vi "Get Bus A Data.vi"(5 "Component ID":u8, 7 "FPGA Interface":refnum<class "FPGA Interface.lvclass">, 8 "error in (no error)":errorcluster, 11 "Bus Monitor in":refnum<class "Bus Monitor.lvclass">) -> (0 "error out":errorcluster, 3 "Bus Monitor out":refnum<class "Bus Monitor.lvclass">)   [LabVIEW 2020, in "BCI-1553 API.lvlib" / "Bus Monitor.lvclass"]
doc: "Retrieves the entire command list for Bus A and parses out a list of command words and data pointer words that are resorted into chronological order."
uses:
  Bus Monitor.lvclass
  Dependencies/FPGA Interface/FPGA Interface.lvclass
  Bus Monitor.lvclass/Bus Monitor.ctl
  Dependencies/Registry/Registry.lvclass/Registry.ctl
  Dependencies/Registry/Registry.lvclass
panel:
  out "Data 2":u16=1 format="%.0x"
  out "Data 1":u16=1 format="%.0x"
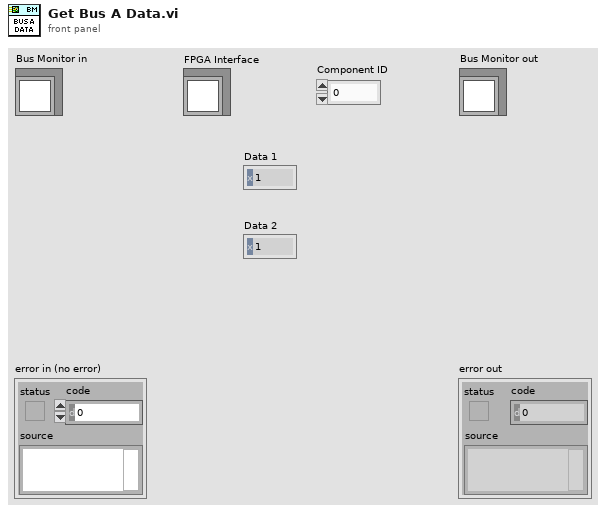
[diagram p1: front panel]
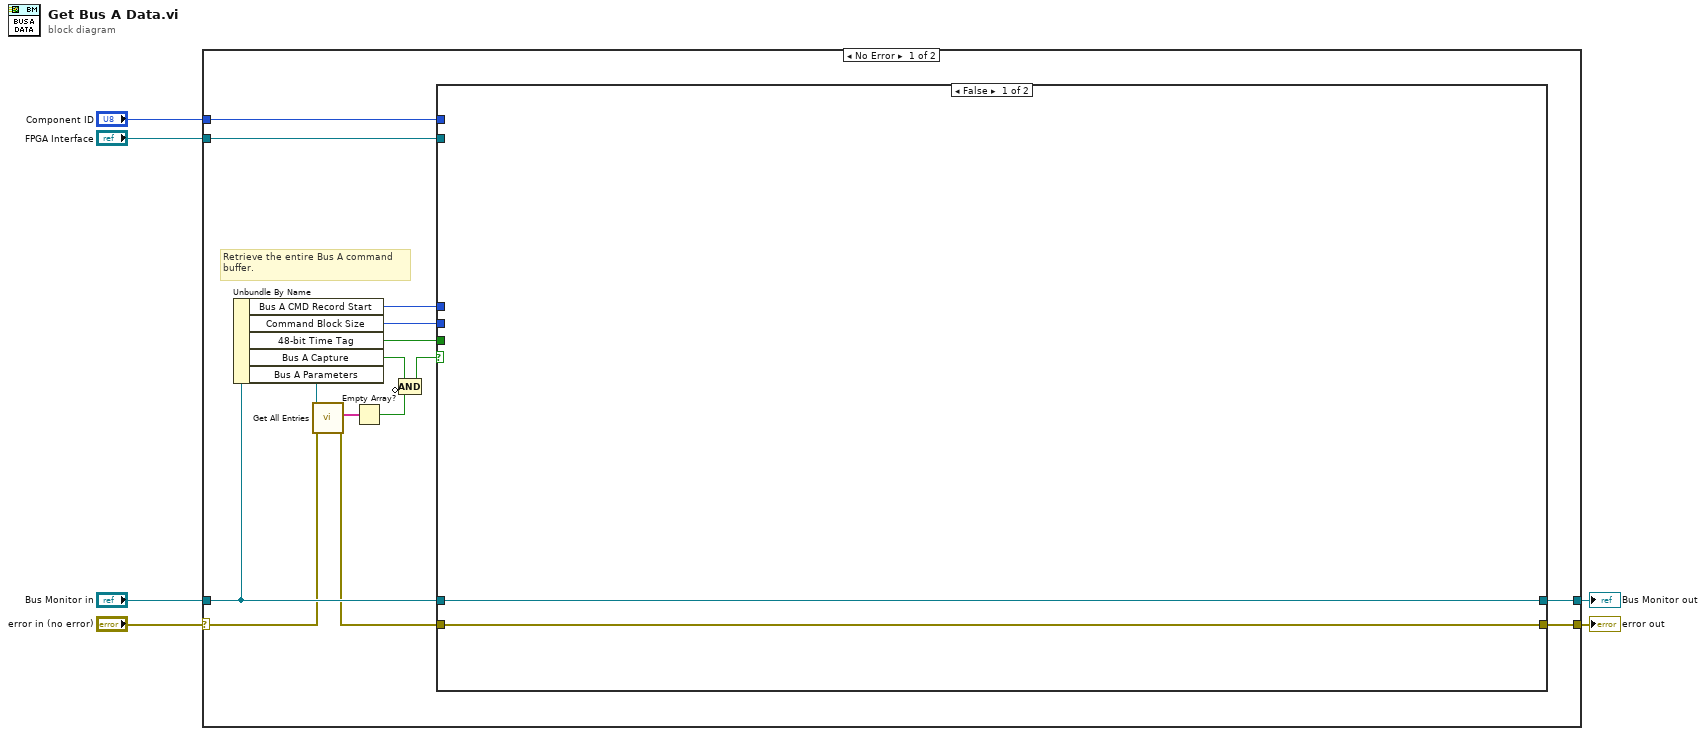
[diagram p0: block diagram]
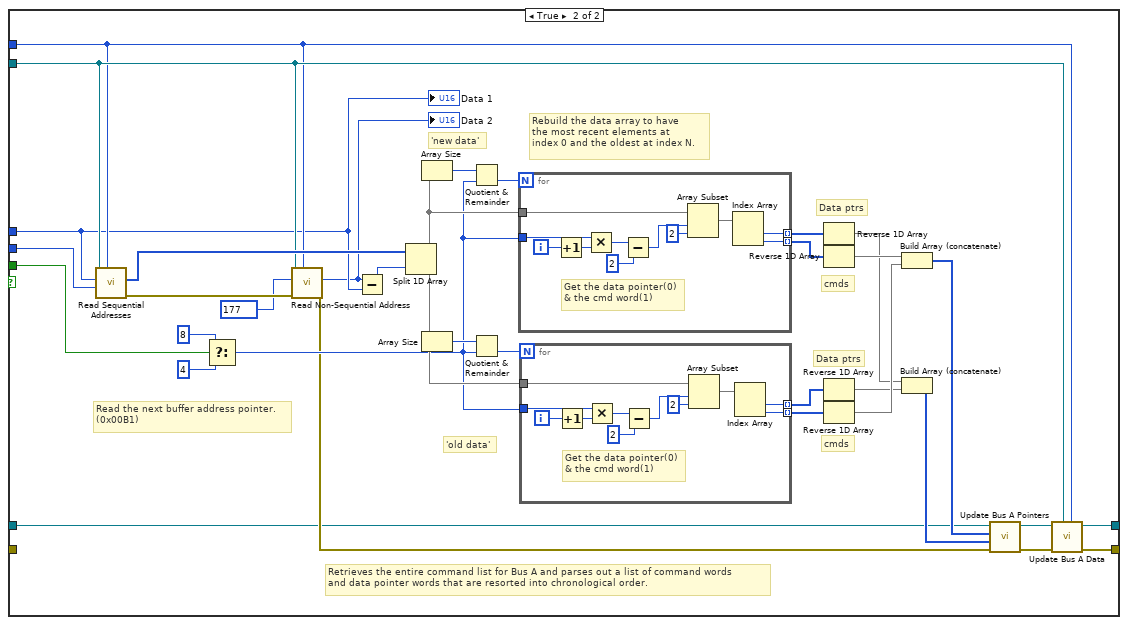
[diagram p2: hidden frame]
diagram:
  n1 = case shown="No Error" "error in (no error)" {
    selector: "error in (no error)" -> [w8 w82]
    tunnel: [w19 w82] -> w5
    tunnel: [w20 w81] -> w3
    tunnel: "Bus Monitor in" -> [w16 w81]
    tunnel: "FPGA Interface" -> [w18 _]
    tunnel: "Component ID" -> [w17 _]
    frame No Error {
      # "Retrieve the entire Bus A command\nbuffer."
      n2 = Unbundle By Name(w16) -> ("Bus A CMD Record Start"=w14:u16, "Command Block Size"=w15:u16, "48-bit Time Tag"=w21:bool, "Bus A Capture"=w13:bool, "Bus A Parameters"=w11:refnum<class "Registry.lvclass">)
      n3 = call "Get All Entries.vi"("error in (no error)"=w8, "Registry in"=w11) -> ("error out"=w7:errorcluster, "Keys"=w10:string[])  [unwired: 7 in, 1 out]
      n4 = Empty Array?(array=w10) -> (empty?=w9:bool)
      n5 = Compound Arithmetic op=AND(w13, invert w9) -> (w12:bool)
      n6 = case shown="False" w12 {
        tunnel: w21 -> [_ w54]
        tunnel: [w23 w32] -> w20
        tunnel: [w22 w30] -> w19
        tunnel: w18 -> [_ w29]
        tunnel: w17 -> [_ w28]
        tunnel: w16 -> [w23 w27]
        tunnel: w15 -> [_ w26]
        tunnel: w14 -> [_ w25]
        tunnel: w7 -> [w22 _]
        frame False {
        }
        frame True {
          # "Retrieves the entire command list for Bus A and parses out a list of command words\nand data pointer words that are resorted into chronological order."
          # "'new data'"
          # "'old data'"
          # "cmds"
          # "Data ptrs"
          # "cmds"
          # "Data ptrs"
          # "Rebuild the data array to have\nthe most recent elements at\nindex 0 and the oldest at index N."
          # "Read the next buffer address pointer.\n(0x00B1)"
          n7 = call-dynamic "Read Sequential Addresses.vi"("Target IC (1-8)"=w28, "Addresses to Read"=w26, "Starting Address"=w25, "FPGA Interface in"=w29) -> ("error out"=w58:errorcluster, "Data"=w55:u16[])  [unwired: 6 in]
          n8 = Select(t=8, s=w54, f=4) -> (s? t:f=w44:i32)
          n9 = call-dynamic "Read Non-Sequential Address.vi"("Target IC (1-8)"=w28, "error in (no error)"=w58, "Address"=u16 177 ("Numeric"), "FPGA Interface in"=w29) -> ("error out"=w36:errorcluster, "Data"=w24:u16)  [unwired: 6 in]
          "Data 2" <- w24
          n10 = Subtract(x=w24, y=w25) -> (x-y=w56:u16)
          n11 = Split 1D Array(array=w55, index=w56) -> (first subarray=w48:u16[], second subarray=w45:u16[])
          n12 = Array Size(array=w48) -> (size(s)=w50:i32)
          n13 = Array Size(array=w45) -> (size(s)=w51:i32)
          n14 = Quotient & Remainder(x=w50, y=w44) -> (floor(x/y)=w49:i32)  [unwired: 1 out]
          n15 = Quotient & Remainder(x=w51, y=w44) -> (floor(x/y)=w46:i32)  [unwired: 1 out]
          n16 = for {
            N: w49 -> [_]
            tunnel: w48 -> [w80]
            tunnel: w44 -> [w79]
            tunnel: [w71] -> w47 mode=indexing
            tunnel: [w70] -> w43 mode=indexing
            i -> [w77]
            # "Get the data pointer(0)\n& the cmd word(1)"
            n17 = Increment(x=w77) -> (x+1=w76:i32)
            n18 = Multiply(x=w79, y=w76) -> (x*y=w75:i32)
            n19 = Subtract(x=w75, y=2 ("length")) -> (x-y=w73:i32)
            n20 = Array Subset(array=w80, index=w73, length=2) -> (w72:u16[])
            n21 = Index Array(array=w72) -> (element #1=w71:u16, element #2=w70:u16)  [unwired: 2 in]
          }
          n22 = for {
            N: w46 -> [_]
            tunnel: w45 -> [w69]
            tunnel: w44 -> [w68]
            tunnel: [w60] -> w42 mode=indexing
            tunnel: [w59] -> w41 mode=indexing
            i -> [w66]
            # "Get the data pointer(0)\n& the cmd word(1)"
            n23 = Increment(x=w66) -> (x+1=w65:i32)
            n24 = Multiply(x=w68, y=w65) -> (x*y=w64:i32)
            n25 = Subtract(x=w64, y=2 ("length")) -> (x-y=w62:i32)
            n26 = Array Subset(array=w69, index=w62, length=2) -> (w61:u16[])
            n27 = Index Array(array=w61) -> (element #1=w60:u16, element #2=w59:u16)  [unwired: 2 in]
          }
          n28 = Reverse 1D Array(array=w47) -> (reversed array=w38:u16[])
          n29 = Reverse 1D Array(array=w43) -> (reversed array=w39:u16[])
          n30 = Reverse 1D Array(array=w42) -> (reversed array=w37:u16[])
          n31 = Reverse 1D Array(array=w41) -> (reversed array=w40:u16[])
          n32 = Build Array (concatenate)(w39, w40) -> (w35:u16[])
          n33 = Build Array (concatenate)(w38, w37) -> (w34:u16[])
          n34 = call "Update Bus A Pointers.vi"("error in (no error)"=w36, "Data Pointers"=w34, "Command Words"=w35, "Bus Monitor in"=w27) -> ("error out"=w31:errorcluster, "Bus Monitor out"=w33:refnum<class "Bus Monitor.lvclass">)  [unwired: 6 in]
          n35 = call "Update Bus A Data.vi"("Component ID"=w28, "FPGA Interface"=w29, "error in (no error)"=w31, "Bus Monitor in"=w33) -> ("error out"=w30:errorcluster, "Bus Monitor out"=w32:refnum<class "Bus Monitor.lvclass">)  [unwired: 6 in]
          "Data 1" <- w25
        }
      }
    }
    frame Error {
    }
  }
  "error out" <- w5
  "Bus Monitor out" <- w3
